vi "Teleop.vi"(10 "Match Info":T2={"Autonomous Elapsed Seconds"=0.0, "TeleOp Elapsed Seconds"=0.0, "Disabled Elapsed Seconds"=0.0, "Visited Autonomous"=FALSE, "Visited TeleOp"=FALSE, "Visited Disabled"=FALSE, "Autonomous Settings"={"Autonomous Style"=enum."Independent", "VI Refnum"=refnum}}, 11 "Call Context":T3) -> ()   [LabVIEW 2014]
doc: "This VI is called for each TeleOp packet received from the DS where the robot is not disabled. It is often used to read from the joysticks and update I/O or to update setpoints for timed control loops. It should complete and return within 20 milliseconds or it may miss DS packets."
uses:
  <vilib>/Rock Robotics/WPI/DriverStation/WPI_DriverStationDerivedRobotMode.ctl
  <vilib>/Rock Robotics/WPI/DriverStation/WPI_DriverStationMatch Info.ctl
  <vilib>/Rock Robotics/WPI/Solenoid/WPI_SolenoidValue.ctl
  <vilib>/Rock Robotics/Network Tables/SD Read Boolean.vi
  <vilib>/Rock Robotics/Network Tables/SD Read Number.vi
  <vilib>/Rock Robotics/Network Tables/SD Write Number.vi
  <vilib>/Rock Robotics/WPI/Joystick/WPI_JoystickGetSetRefNum.vi
  <vilib>/Rock Robotics/WPI/Solenoid/WPI_SolenoidSetEnum.vi
  <vilib>/Rock Robotics/Network Tables/SD Write Boolean Array.vi
  <vilib>/Rock Robotics/Network Tables/SD Write Numeric Array.vi
  <vilib>/Rock Robotics/WPI/RobotDrive/WPI_RobotDriveGetSetRefNum.vi
  <vilib>/addons/control/pid/pid.llb/PID (DBL).vi
  <vilib>/Rock Robotics/WPI/RobotDrive/WPI_RobotDriveMecanumDrive_Cartesian.vi
  <vilib>/addons/control/pid/NI_PID_pid.lvlib
panel:
  out "rot/360":dbl
  out "arctan/360":dbl
  out "atan2(y,x)":dbl
  out "x > y?":bool
  out "PV rotate":dbl
  out "SP rotate":dbl
  in  "PID gains 2":T1={"proportional gain (Kc)"=0.025, "integral time (Ti, min)"=0.02, "derivative time (Td, min)"=0.0} {"derivative time (Td, min)" format="%.3f"; "integral time (Ti, min)" format="%.3f"; "proportional gain (Kc)" format="%.3f"}
  out "Boolean":bool=TRUE
  out "Header 2":dbl
  out "PID Output":dbl format="%.2f"
  out "Angle":dbl
  in  "STRAIGHT PID  2":T1={"proportional gain (Kc)"=0.025, "integral time (Ti, min)"=0.02, "derivative time (Td, min)"=0.0} {"derivative time (Td, min)" format="%.3f"; "integral time (Ti, min)" format="%.3f"; "proportional gain (Kc)" format="%.3f"}
  out "X 2":dbl
  out "Y 2":dbl
  out "R 2":dbl
  out "X":dbl
  out "Y":dbl
  out "R":dbl
  out "Header":dbl
  in  "PID gains":T1={"proportional gain (Kc)"=1.0, "integral time (Ti, min)"=0.01, "derivative time (Td, min)"=0.0} {"derivative time (Td, min)" format="%.3f"; "integral time (Ti, min)" format="%.3f"; "proportional gain (Kc)" format="%.3f"}
  in  "STRAIGHT PID":T1={"proportional gain (Kc)"=1.0, "integral time (Ti, min)"=0.01, "derivative time (Td, min)"=0.0} {"derivative time (Td, min)" format="%.3f"; "integral time (Ti, min)" format="%.3f"; "proportional gain (Kc)" format="%.3f"}
  out "Sample Slider 0":dbl(slide) scale=0.0..5.0
  out "Sample Boolean 1":bool
  out "Sample Boolean 0":bool
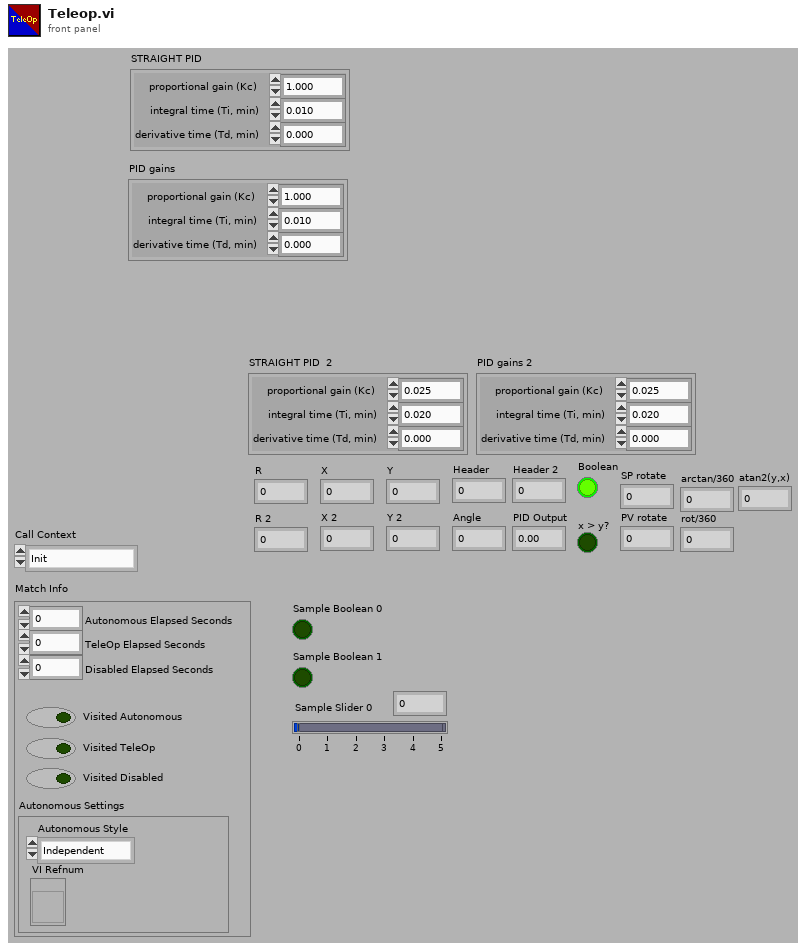
[diagram p1: front panel]
types:
  T1 = cluster{"proportional gain (Kc)":dbl, "integral time (Ti, min)":dbl, "derivative time (Td, min)":dbl}
  T2 = typedef "WPI_DriverStationMatch Info.ctl" = cluster{"Autonomous Elapsed Seconds":dbl, "TeleOp Elapsed Seconds":dbl, "Disabled Elapsed Seconds":dbl, "Visited Autonomous":bool, "Visited TeleOp":bool, "Visited Disabled":bool, "Autonomous Settings":cluster{"Autonomous Style":enum16{"Iterative", "Independent"}, "VI Refnum":refnum<vi>}}
  T3 = typedef "WPI_DriverStationDerivedRobotMode.ctl" = enum16{"Init", "Execute", "Stop"}
  T4 = typedef "WPI_SolenoidValue.ctl" = enum16{"Off", "On", "Forward", "Reverse"}
  T5 = typedef "WPI_JoystickDevRef.ctl" = cluster{"Device":T6}
  T6 = typedef "WPI_JoystickDeviceEnum.ctl" = enum16{"USB 0", "USB 1", "USB 2", "USB 3", "USB 4", "USB 5"}
  T7 = typedef "WPI_GyroDevRef.ctl" = cluster{"DevStatus":errorcluster, "Analog Module":T8, "Analog Channel":T9, "Offset":dbl, "Gain (VoltsPerDegree/Second)":dbl}
  T8 = typedef "FPGA_TypedefAnalogModule.ctl" = enum16{"Controller 1"}
  T9 = typedef "FPGA_AIChannel.ctl" = enum8{"AI 0", "AI 1", "AI 2", "AI 3", "AI MXP 0", "AI MXP 1", "AI MXP 2", "AI MXP 3", "Invalid"}
  T10 = typedef "WPI_RobotDriveDevRef.ctl" = cluster{"DevStatus":errorcluster, "Motors[]":T11[], "Square Inputs":bool, "Max Output":dbl}
  T11 = typedef "WPI_MotorControlDeviceRef.ctl" = cluster{"DeviceStatus":errorcluster, "Type":T12, "PWM":cluster{"Controller":T13, "PWM Channel":T14, "DeadBand":T15}, "CAN":cluster{"Device Number":u8, "Control Mode":T16, "Semaphore":T17, "Max Vout":dbl, "TalonSRX Control Mode":T18}, "Invert":bool, "TransformRef":T19, "InvTransformRef":T19}
  T12 = typedef "WPI_MotorControlType.ctl" = enum16{"PWM", "CAN", "CANTalonSRX"}
  T13 = typedef "FPGA_TypedefDigitalModule.ctl" = enum16{"Controller 1"}
  T14 = typedef "FPGA_DIOPWMChannel.ctl" = enum8{"PWM 0", "PWM 1", "PWM 2", "PWM 3", "PWM 4", "PWM 5", "PWM 6", "PWM 7", "PWM 8", "PWM 9", "PWM MXP 0", "PWM MXP 1", "PWM MXP 2", "PWM MXP 3", "PWM MXP 4", "PWM MXP 5", "PWM MXP 6", "PWM MXP 7", "PWM MXP 8", "PWM MXP 9", "Invalid"}
  T15 = typedef "WPI_PWMDeadband.ctl" = cluster{"Name":string, "maxPositivePwm":i32, "minPositivePwm":i32, "centerPwm":i32, "maxNegativePwm":i32, "minNegativePwm":i32, "angularRange":u16}
  T16 = typedef "WPI_CANJaguar_ControlMode.ctl" = enum8{"Percent VBus", "Current", "Speed", "Position", "Voltage"}
  T17 = typedef "Semaphore RefNum" = refnum<k1>
  T18 = typedef "WPI_CANTalonSRX_APIControlMode.ctl" = enum8{"Percent VBus", "Speed", "Position", "Slave", "Unchanged / Invalid"}
  T19 = typedef "WPI_PWMTransform_ConPane.ctl" = refnum<vi>
  T20 = typedef "WPI_SolenoidDevRef.ctl" = cluster{"DevStatus":errorcluster, "Pneumatics Control Module":u8, "Forward Solenoid Channel":T21, "Reverse Solenoid Channel":T21}
  T21 = typedef "WPI_SolenoidChannel.ctl" = enum8{"Solenoid 0", "Solenoid 1", "Solenoid 2", "Solenoid 3", "Solenoid 4", "Solenoid 5", "Solenoid 6", "Solenoid 7", "Invalid"}
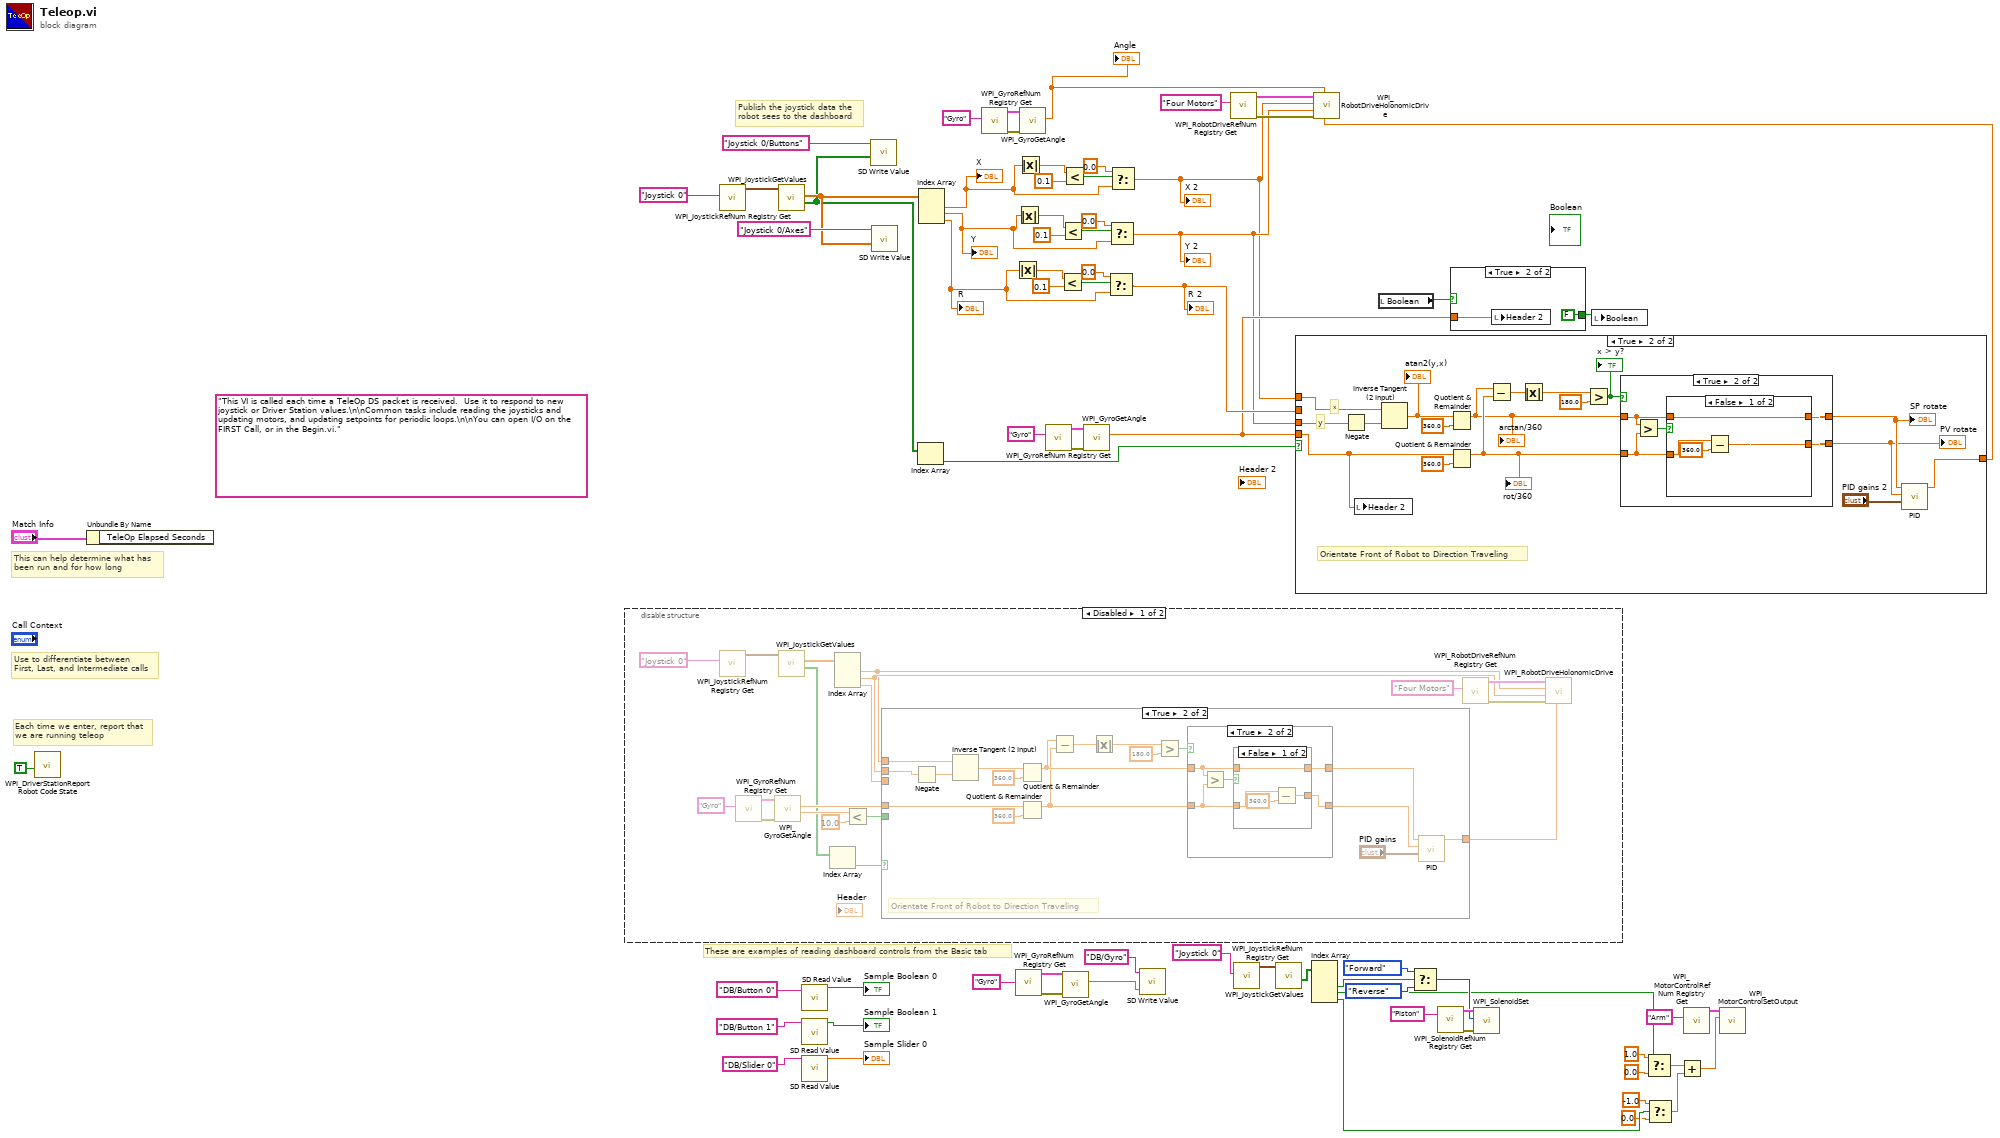
[diagram p0: block diagram]
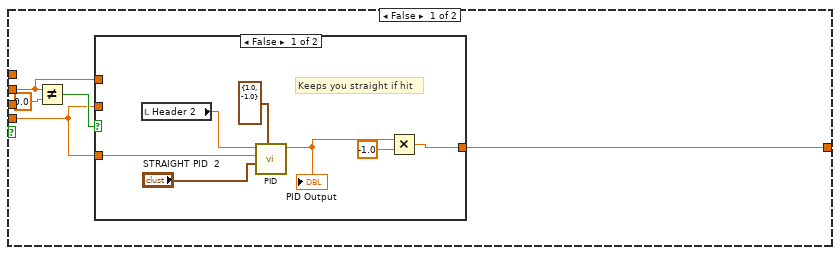
[diagram p2: hidden frame]
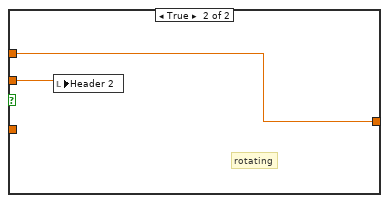
[diagram p3: hidden frame]
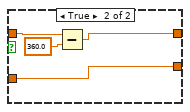
[diagram p5: hidden frame]
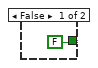
[diagram p6: hidden frame]
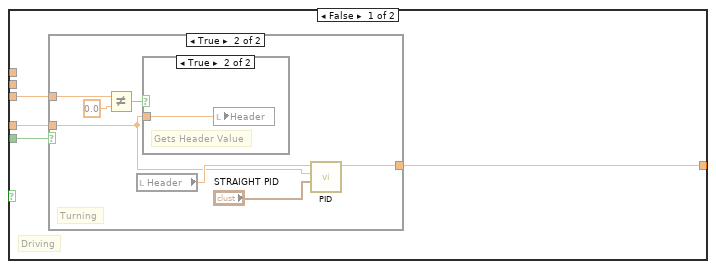
[diagram p7: hidden frame]
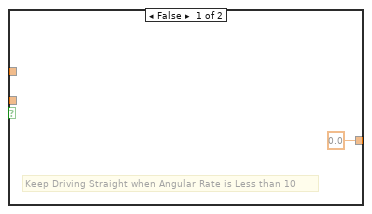
[diagram p8: hidden frame]
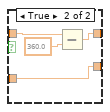
[diagram p11: hidden frame]
diagram:
  (unwired) "This VI is called each time a TeleOp DS packet is received.  Use it to respond to new joystick or Driver Station values.\n\nCommon tasks include reading the joysticks and updating motors, and updating setpoints for periodic loops.\n\nYou can open I/O on the FIRST Call, or in the Begin.vi."
  # "Publish the joystick data the\nrobot sees to the dashboard"
  # "These are examples of reading dashboard controls from the Basic tab"
  # "Each time we enter, report that\nwe are running teleop"
  # "Use to differentiate between\nFirst, Last, and Intermediate calls"
  # "This can help determine what has\nbeen run and for how long"
  n1 = call <vilib>:"WPI_DriverStationReport Robot Code State.vi"("TeleOp"=TRUE ("Autonomous")) -> ()  [unwired: 10 in, 1 out]
  n2 = Unbundle By Name("Match Info") -> ()  [unwired: 1 out]
  n3 = disable-structure shown="Disabled" {
    frame Disabled {
      n4 = call <vilib>:"WPI_JoystickRefNum Registry Get.vi"("refnum name"="Joystick 0") -> ("JoystickDevRef"=w88:T5)  [unwired: 1 in, 9 out]
      n5 = call <vilib>:"WPI_GyroRefNum Registry Get.vi"("refnum name"="Gyro") -> ("error out"=w83:errorcluster, "GyroDevRef"=w86:T7)  [unwired: 9 in]
      n6 = call <vilib>:"WPI_GyroGetAngle.vi"("error in (no error)"=w83, "GyroDevRef"=w86) -> ("Angular Rate"=w79:dbl, "Angle"=w84:dbl)  [unwired: 6 in, 2 out]
      n7 = call <vilib>:"WPI_JoystickGetValues.vi"("JoystickDevRef"=w88) -> ("Buttons"=w77:bool[], "Axes"=w89:dbl[])  [unwired: 6 in, 3 out]
      n8 = Index Array(array=w77) -> (element=w76:bool)  [unwired: 1 in]
      n9 = Index Array(array=w89) -> (element #1=w74:dbl, element #2=w75:dbl, element #3=w81:dbl)  [unwired: 3 in]
      n10 = Less?(x=w79, y=10.0) -> (x < y?=w80:bool)
      n11 = case shown="True" w76 {
        tunnel: w84 -> [w96 w117]
        tunnel: [w95 w106] -> w82
        tunnel: w81 -> [w94 _]
        tunnel: w80 -> [w93 _]
        tunnel: w75 -> [_ w121]
        tunnel: w74 -> [_ w116]
        frame False {
          # "Driving"
          n12 = case shown="True" w93 {
            tunnel: w96 -> [_ w98]
            tunnel: [0.0 ("output") w104] -> w95
            tunnel: w94 -> [_ w103]
            frame False {
              # "Keep Driving Straight when Angular Rate is Less than 10"
            }
            frame True {
              # "Turning"
              n13 = Not Equal?(x=w103, y=0.0) -> (x != y?=w100:bool)
              n14 = local read "Header"() -> (w102:dbl)
              n15 = case shown="True" w100 {
                tunnel: w98 -> [_ w105]
                frame False {
                }
                frame True {
                  # "Gets Header Value"
                  n16 = local write "Header"(w105) -> ()
                }
              }
              n17 = call-poly <vilib>:"PID.vi"("PID gains"="STRAIGHT PID", "process variable"=w98, "setpoint"=w102) -> ("output"=w104:dbl)  [unwired: 7 in, 1 out]
            }
          }
        }
        frame True {
          # "Orientate Front of Robot to Direction Traveling"
          n18 = Negate(x=w121) -> (-x=w122:dbl)
          n19 = Inverse Tangent (2 Input)(1:w122, 2:w116) -> (0:w120:dbl)
          n20 = Quotient & Remainder(x=w120, y=360.0) -> (x-y*floor(x/y)=w112:dbl)  [unwired: 1 out]
          n21 = Quotient & Remainder(x=w117, y=360.0) -> (x-y*floor(x/y)=w111:dbl)  [unwired: 1 out]
          n22 = Subtract(x=w112, y=w111) -> (x-y=w115:dbl)
          n23 = Absolute Value(x=w115) -> (abs(x)=w114:dbl)
          n24 = Greater?(x=w114, y=180.0) -> (0:w110:bool)
          n25 = case shown="True" w110 {
            tunnel: w112 -> [w124 w128]
            tunnel: w111 -> [w123 w127]
            tunnel: [w124 w126] -> w108
            tunnel: [w123 w125] -> w107
            frame False {
            }
            frame True {
              n26 = Greater?(x=w128, y=w127) -> (0:w129:bool)
              n27 = case shown="False" w129 {
                tunnel: w128 -> [w133 w136]
                tunnel: w127 -> [w132 w135]
                tunnel: [w133 w137] -> w126
                tunnel: [w130 w135] -> w125
                frame False {
                  n28 = Subtract(x=w132, y=360.0) -> (x-y=w130:dbl)
                }
                frame True {
                  n29 = Subtract(x=w136, y=360.0) -> (x-y=w137:dbl)
                }
              }
            }
          }
          n30 = call-poly <vilib>:"PID.vi"("PID gains"="PID gains", "process variable"=w107, "setpoint"=w108) -> ("output"=w106:dbl)  [unwired: 7 in, 1 out]
        }
      }
      n31 = call <vilib>:"WPI_RobotDriveRefNum Registry Get.vi"("refnum name"="Four Motors") -> ("error out"=w91:errorcluster, "RobotDriveDevRef"=w92:T10)  [unwired: 9 in]
      n32 = call-poly <vilib>:"WPI_RobotDriveHolonomicDrive.vi"("Rotation"=w82, "error in (no error)"=w91, "Y"=w75, "X"=w74, "RobotDriveDevRef"=w92) -> ()  [unwired: 4 in, 3 out]
    }
    frame Enabled {
    }
  }
  n33 = call <vilib>:"WPI_JoystickRefNum Registry Get.vi"("refnum name"="Joystick 0") -> ("JoystickDevRef"=w49:T5)  [unwired: 1 in, 9 out]
  n34 = call <vilib>:"WPI_JoystickGetValues.vi"("JoystickDevRef"=w49) -> ("Buttons"=w14:bool[], "Axes"=w44:dbl[])  [unwired: 6 in, 3 out]
  n35 = call-poly <vilib>:"SD Read Value.vi"("Name"="DB/Button 0" ("refnum name")) -> ("Boolean"=→"Sample Boolean 0":bool)  [unwired: 8 in, 2 out]
  n36 = call-poly <vilib>:"SD Read Value.vi"("Name"="DB/Button 1" ("refnum name")) -> ("Boolean"=→"Sample Boolean 1":bool)  [unwired: 8 in, 2 out]
  n37 = call-poly <vilib>:"SD Read Value.vi"("Name"="DB/Slider 0" ("refnum name")) -> ("Numeric"=→"Sample Slider 0":dbl)  [unwired: 8 in, 2 out]
  n38 = call-poly <vilib>:"SD Write Value.vi"("Boolean Array"=w14, "Name"="Joystick 0/Buttons") -> ()  [unwired: 8 in, 2 out]
  n39 = call-poly <vilib>:"SD Write Value.vi"("Numeric Array"=w44, "Name"="Joystick 0/Axes") -> ()  [unwired: 8 in, 2 out]
  n40 = Index Array(array=w14) -> (element=w15:bool)  [unwired: 1 in]
  n41 = Index Array(array=w44) -> (element #1=w22:dbl, element #2=w24:dbl, element #3=w23:dbl)  [unwired: 3 in]
  "R" <- w23
  "Y" <- w24
  "X" <- w22
  n42 = call <vilib>:"WPI_GyroRefNum Registry Get.vi"("refnum name"="Gyro") -> ("error out"=w36:errorcluster, "GyroDevRef"=w38:T7)  [unwired: 9 in]
  n43 = Absolute Value(x=w23) -> (abs(x)=w28:dbl)
  n44 = call <vilib>:"WPI_GyroRefNum Registry Get.vi"("refnum name"="Gyro") -> ("error out"=w53:errorcluster, "GyroDevRef"=w54:T7)  [unwired: 9 in]
  n45 = Absolute Value(x=w24) -> (abs(x)=w29:dbl)
  n46 = Absolute Value(x=w22) -> (abs(x)=w42:dbl)
  n47 = call <vilib>:"WPI_GyroGetAngle.vi"("error in (no error)"=w36, "GyroDevRef"=w38) -> ("Angle"=w35:dbl)  [unwired: 6 in, 3 out]
  "Angle" <- w35
  n48 = call <vilib>:"WPI_GyroRefNum Registry Get.vi"("refnum name"="Gyro") -> ("error out"=w16:errorcluster, "GyroDevRef"=w17:T7)  [unwired: 9 in]
  n49 = Less?(x=w28, y=0.1) -> (x < y?=w26:bool)
  n50 = Less?(x=w29, y=0.1) -> (x < y?=w31:bool)
  n51 = Less?(x=w42, y=0.1) -> (x < y?=w40:bool)
  n52 = call <vilib>:"WPI_GyroGetAngle.vi"("error in (no error)"=w53, "GyroDevRef"=w54) -> ("Angle"=w56:dbl)  [unwired: 6 in, 3 out]
  n53 = call <vilib>:"WPI_GyroGetAngle.vi"("error in (no error)"=w16, "GyroDevRef"=w17) -> ("Angle"=w20:dbl)  [unwired: 6 in, 3 out]
  n54 = Select(t=0.0, s=w26, f=w23) -> (s? t:f=w21:dbl)
  "R 2" <- w21
  n55 = Select(t=0.0, s=w31, f=w24) -> (s? t:f=w13:dbl)
  "Y 2" <- w13
  n56 = Select(t=0.0, s=w40, f=w22) -> (s? t:f=w12:dbl)
  "X 2" <- w12
  n57 = call-poly <vilib>:"SD Write Value.vi"("Numeric"=w56, "Name"="DB/Gyro") -> ()  [unwired: 8 in, 2 out]
  n58 = call <vilib>:"WPI_RobotDriveRefNum Registry Get.vi"("refnum name"="Four Motors") -> ("error out"=w46:errorcluster, "RobotDriveDevRef"=w45:T10)  [unwired: 9 in]
  n59 = call <vilib>:"WPI_JoystickRefNum Registry Get.vi"("refnum name"="Joystick 0") -> ("JoystickDevRef"=w58:T5)  [unwired: 1 in, 9 out]
  n60 = call <vilib>:"WPI_JoystickGetValues.vi"("JoystickDevRef"=w58) -> ("Buttons"=w59:bool[])  [unwired: 6 in, 4 out]
  n61 = case shown="True" w15 {
    tunnel: [w142 w153] -> w33
    tunnel: w21 -> [w139 _]
    tunnel: w20 -> [w138 w152]
    tunnel: w13 -> [_ w160]
    tunnel: w12 -> [_ w159]
    frame False {
      n62 = Not Equal?(x=w139, y=0.0) -> (x != y?=w140:bool)
      n63 = case shown="False" w140 {
        tunnel: [w148 w151] -> w142
        tunnel: w138 -> [w149 _]
        tunnel: w138 -> [_ w150]
        tunnel: w139 -> [_ w151]
        frame False {
          # "Keeps you straight if hit"
          n64 = local read "Header 2"() -> (w145:dbl)
          n65 = call-poly <vilib>:"PID.vi"("output range"=cluster{"output high":dbl, "output low":dbl} {"output high"=1.0, "output low"=-1.0}, "PID gains"="STRAIGHT PID  2", "process variable"=w149, "setpoint"=w145) -> ("output"=w144:dbl)  [unwired: 6 in, 1 out]
          "PID Output" <- w144
          n66 = Multiply(x=w144, y=-1.0) -> (x*y=w148:dbl)
        }
        frame True {
          # "rotating"
          n67 = local write "Header 2"(w150) -> ()
        }
      }
    }
    frame True {
      # "y"
      # "x"
      # "Orientate Front of Robot to Direction Traveling"
      n68 = Negate(x=w160) -> (-x=w161:dbl)
      n69 = local write "Header 2"(w152) -> ()
      n70 = Inverse Tangent (2 Input)(1:w161, 2:w159) -> (0:w162:dbl)
      "atan2(y,x)" <- w162
      n71 = Quotient & Remainder(x=w162, y=360.0) -> (x-y*floor(x/y)=w156:dbl)  [unwired: 1 out]
      "arctan/360" <- w156
      n72 = Quotient & Remainder(x=w152, y=360.0) -> (x-y*floor(x/y)=w157:dbl)  [unwired: 1 out]
      "rot/360" <- w157
      n73 = Subtract(x=w156, y=w157) -> (x-y=w165:dbl)
      n74 = Absolute Value(x=w165) -> (abs(x)=w166:dbl)
      n75 = Greater?(x=w166, y=180.0) -> (0:w158:bool)
      "x > y?" <- w158
      n76 = case shown="True" w158 {
        tunnel: w156 -> [w170 w174]
        tunnel: w157 -> [w169 w173]
        tunnel: [w170 w172] -> w155
        tunnel: [w169 w171] -> w154
        frame False {
        }
        frame True {
          n77 = Greater?(x=w174, y=w173) -> (0:w175:bool)
          n78 = case shown="False" w175 {
            tunnel: w174 -> [w179 w182]
            tunnel: w173 -> [w178 w181]
            tunnel: [w179 w183] -> w172
            tunnel: [w176 w181] -> w171
            frame False {
              n79 = Subtract(x=w178, y=360.0) -> (x-y=w176:dbl)
            }
            frame True {
              n80 = Subtract(x=w182, y=360.0) -> (x-y=w183:dbl)
            }
          }
        }
      }
      "SP rotate" <- w155
      "PV rotate" <- w154
      n81 = call-poly <vilib>:"PID.vi"("PID gains"="PID gains 2", "process variable"=w154, "setpoint"=w155) -> ("output"=w153:dbl)  [unwired: 7 in, 1 out]
    }
  }
  n82 = Index Array(array=w59) -> (element #2=w51:bool, element #3=w9:bool, element #4=w6:bool)  [unwired: 4 in, 1 out]
  n83 = call-poly <vilib>:"WPI_RobotDriveHolonomicDrive.vi"("Rotation"=w33, "Gyro Angle"=w35, "error in (no error)"=w46, "Y"=w13, "X"=w12, "RobotDriveDevRef"=w45) -> ()  [unwired: 3 in, 3 out]
  n84 = local read "Boolean"() -> (w19:bool)
  n85 = Select(t=WPI_SolenoidValue."Forward" ("Value"), s=w51, f=WPI_SolenoidValue."Reverse" ("Value")) -> (s? t:f=w62:T4)
  n86 = call <vilib>:"WPI_SolenoidRefNum Registry Get.vi"("refnum name"="Piston") -> ("error out"=w63:errorcluster, "SolenoidDevRef"=w64:T20)  [unwired: 9 in]
  n87 = case shown="True" w19 {
    tunnel: w20 -> [_ w186]
    tunnel: [FALSE FALSE] -> w18
    frame False {
    }
    frame True {
      n88 = local write "Header 2"(w186) -> ()
    }
  }
  n89 = call-poly <vilib>:"WPI_SolenoidSet.vi"("error in (no error)"=w63, "Value"=w62, "SolenoidDevRef"=w64) -> ()  [unwired: 7 in, 2 out]
  n90 = local write "Boolean"(w18) -> ()
  n91 = Select(t=1.0, s=w9, f=0.0) -> (s? t:f=w3:dbl)
  n92 = Select(t=-1.0, s=w6, f=0.0) -> (s? t:f=w2:dbl)
  n93 = Add(x=w3, y=w2) -> (x+y=w1:dbl)
  n94 = call <vilib>:"WPI_MotorControlRefNum Registry Get.vi"("refnum name"="Arm") -> ("MotorControlDevRef"=w10:T11)  [unwired: 9 in, 1 out]
  n95 = call <vilib>:"WPI_MotorControlSetOutput.vi"("Output"=w1, "MotorControlDevRef"=w10) -> ()  [unwired: 7 in, 3 out]
